vi "Instrument Identifiers.vi"(0 "VISA resource name":refnum<visa-resource-name>, 1 "Unit Address (1)":u8=1 min=1 max=254, 11 "error in (no error)":errorcluster) -> (3 "Instrument\nIdentity":i16 format="%x", 4 "VISA resource name out":refnum<visa-resource-name>, 6 "Instrument Version\nnumber":u16 format="%x", 10 "Company ID":u16, 14 "Customer Defined\nID (0)":u16, 15 "error out":errorcluster)   [LabVIEW 2010, in "Eurotherm 32xx Series.lvlib"]
doc: "This VI returns Instrument Identifiers."
uses:
  <instrlib>/Eurotherm 32xx Series/Eurotherm 32xx Series.lvlib
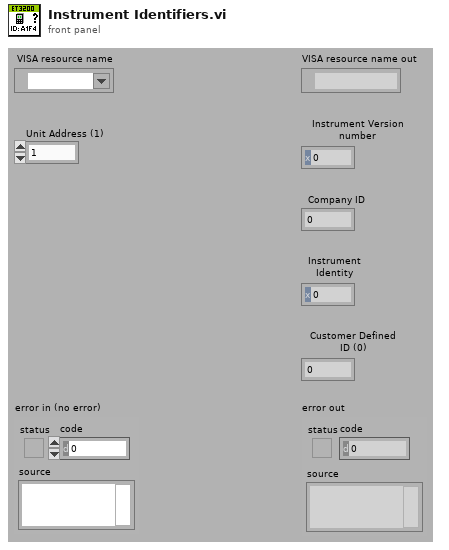
[diagram p1: front panel]
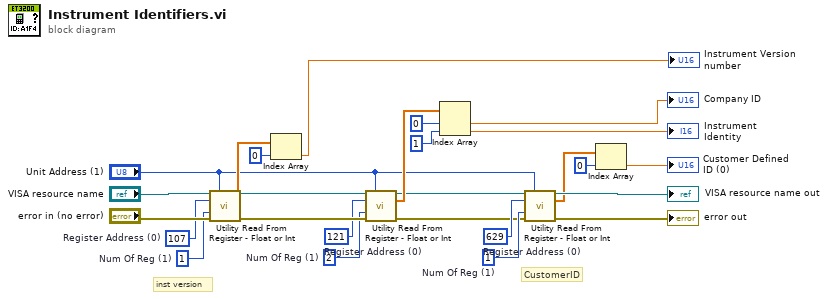
[diagram p0: block diagram]
diagram:
  w11 = u16 629  # Register Address (0)
  w10 = u16 1  # Num Of Reg (1)
  w16 = u16 121  # Register Address (0)
  w17 = u16 107  # Register Address (0)
  w18 = u16 2  # Num Of Reg (1)
  w24 = u16 1  # Num Of Reg (1)
  # "CustomerID"
  # "inst version"
  n1 = call <instrlib>:"Utility Read From Register - Float or Int.vi"("VISA resource name"="VISA resource name", "Unit Address (1)"="Unit Address (1)", "Register Address (0)"=w17, "Num Of Reg (1)"=w24, "error in (no error)"="error in (no error)") -> ("VISA resource name out"=w20:refnum<visa-resource-name>, "Data"=w23:sgl[], "error out"=w19:errorcluster)  [unwired: 8 in]
  n2 = Index Array(array=w23, index=0) -> (element=→"Instrument Version\nnumber":sgl)
  n3 = call <instrlib>:"Utility Read From Register - Float or Int.vi"("VISA resource name"=w20, "Unit Address (1)"="Unit Address (1)", "Register Address (0)"=w16, "Num Of Reg (1)"=w18, "error in (no error)"=w19) -> ("VISA resource name out"=w7:refnum<visa-resource-name>, "Data"=w13:sgl[], "error out"=w6:errorcluster)  [unwired: 8 in]
  n4 = Index Array(array=w13, index #1=0 ("index"), index #2=1 ("index")) -> (element #1=→"Company ID":sgl, element #2=→"Instrument\nIdentity":sgl)
  n5 = call <instrlib>:"Utility Read From Register - Float or Int.vi"("VISA resource name"=w7, "Unit Address (1)"="Unit Address (1)", "Register Address (0)"=w11, "Num Of Reg (1)"=w10, "error in (no error)"=w6) -> ("VISA resource name out"=→"VISA resource name out":refnum<visa-resource-name>, "Data"=w4:sgl[], "error out"=→"error out":errorcluster)  [unwired: 8 in]
  n6 = Index Array(array=w4, index=0) -> (element=→"Customer Defined\nID (0)":sgl)
